vi "HEWH_DSM_CMD.vi"(5 "Temperature":u8=100, 7 "Vacation Days":u8=180, 8 "Heating Mode":T1, 9 "GEA2 Commands and Requests":T2=enum."CMD_WRITE_SETPOINTS") -> (1 "CMD Array":u8[](array[numeric]) format="%x", 2 "Input Data":T5 {"Command" format="%02x"; "Destination" format="%02x"; "Source" format="%02x"})   [LabVIEW 2016]
uses:
  LabVIEW GEA2 Toolkit v1.0.0.0/type defs/Data In.ctl
  Type Definitions/GEA2 Commands.ctl
  Save File/File Setup (Public)/Type Definition/Save File HEWH Heating Control Mode.ctl
  LabVIEW GEA2 Toolkit v1.0.0.0/library/GEA2_Toolkit.lvlib
  Save File/File Setup.lvlib
panel:
  out "element":T3 {"CMD Array" format="%x"; "Destination" format="%x"}
  out "GEA2 Command Cluster":T4(array[cluster])
  out "GEA2 Command Table":string[][](array[string])=[["CMD_WRITE_SETPOINTS", "0x60", "0xA5", "N/A", "Any"], ["RQST_NON_CRIT_VERSION", "0x60", "0x01", "N/A", "Any"], ["RQST_CRIT_VERSION", "0x60", "0x02", "N/A", "Any"], ["RQST_EEPROM_VERSION", "0x60", "0x03", "N/A", "Any"], ["RQST_T2_RESISTANCE", "0x60", "0x10", "N/A", "Any"], ["RQST_T3A_RESISTANCE", "0x60", "0x11", "N/A", "Any"], ["RQST_T3B_RESISTANCE", "0x60", "0x12", "N/A", "Any"], ["RQST_T4_RESISTANCE", "0x60", "0x13", "N/A", "Any"], ["RQST_T5_RESISTANCE", "0x60", "0x14", "N/A", "Any"], ["RQST_IDLB_RESISTANCE", "0x60", "0x15", "N/A", "Any"], ["RQST_MODE_SELECT_RESISTANCE", "0x60", "0x16", "N/A", "Any"], ["RQST_STATUS INFO", "0x60", "0x50", "N/A", "Any"], ["RQST_SS_FAULT_COUNTS", "0x60", "0x53", "N/A", "Any"], ["RQST_OTHER_FAULT_COUNTS", "0x60", "0x54", "N/A", "Any"], ["CMD_CLEAR_FAULT_COUNTS", "0x60", "0x55", "N/A", "Any"], ["RQST_HYPERTERM_OUTPUT_DATA", "0x60", "0x56", "N/A", "Any"], ["RQST_READ_PERSONALITY", "0x60", "0xBC", "N/A", "Any"], ["RQST_DSM_OVERRIDE_STATUS", "0x60", "0xDE", "0x02", "Any"], ["RQST_STATUS_QUERY", "0x60", "0xDE", "0x10", "Any"], ["RQST_HEM_KWH_DATA", "0x60", "0xDE", "0x12", "Any"], ["RQST_SERVICE_ERROR_CODES", "0x60", "0xDE", "0x14", "Any"], ["RQST_OVERRIDE_STATUS", "0x60", "0xDE", "0x17", "Any"], ["CMD_CLEAR_OVERRIDE_STATUS", "0x60", "0xDF", "0x03", "0x40"], ["CMD_CLEAR_ENERGY_USAGE_CTRS", "0x60", "0xDF", "0x07", "0x40"], ["CMD_COMP_OFF", "0x60", "0xF0", "N/A", "Any"], ["CMD_UE_2_SECONDS", "0x60", "0xF3", "N/A", "Any"], ["CMD_LE_2_SECONDS", "0x60", "0xF4", "N/A", "Any"], ["CMD_COMP_ON", "0x60", "0xF5", "N/A", "Any"], ["CMD_HP_RUN_6MIN", "0x60", "0xF6", "N/A", "Any"], ["RQST_TEMP_RANGE", "0x60", "0xF7", "N/A", "Any"], ["RQST_VACATION_RANGE", "0x60", "0xF8", "N/A", "Any"], ["RQST_STD_ELEC_RANGE", "0x60", "0xF9", "N/A", "Any"], ["RQST_WATER_CAPACITY", "0x60", "0xFA", "N/A", "Any"], ["CMD_CANCEL_EEV_POSITION", "0x60", "0xFB", "N/A", "Any"], ["RQST_SUPPORTED_MODES", "0x60", "0xFE", "N/A", "Any"], ["CMD_CONTROL_FAN1", "0x60", "0xF1", "N/A", "Any"], ["CMD_EEV_POSITION", "0x60", "0xFC", "N/A", "Any"], ["CMD_SET_EEV_START_POSITION", "0x60", "E5", "N/A", "Any"], ["CMD_SET_EEV_STOP_POSITION", "0x60", "EA", "N/A", "Any"], ["CMD_UPDATE_DSM_LEVEL", "0x60", "0xDF", "0x00", "0x40"], ["CMD_SET_PID_I_DENOMINATOR", "0x60", "E3", "N/A", "Any"], ["CMD_SET_PID_I_NUMERATOR", "0x60", "E2", "N/A", "Any"], ["RQST_DATA_FROM_MEMORY", "0x60", "0x4E", "N/A", "Any"], ["CMD_OVERRIDE_STATUS_CHANGED", "0x40", "0xDF", "0x02", "0x60"], ["CMD_SET_PID_P_DENOMINATOR", "0x60", "E1", "N/A", "Any"], ["CMD_SET_PID_P_NUMERATOR", "0x60", "E0", "N/A", "Any"], ["CMD_SET_PID_RUN_SH_TARGET", "0x60", "E9", "N/A", "Any"], ["CMD_SET_PID_START_DWELL_TIME", "0x60", "E6", "N/A", "Any"], ["CMD_SET_PID_TRANSITION_TIME", "0x60", "E8", "N/A", "Any"], ["CMD_SET_PID_TRANS_SH_TARGET", "0x60", "E7", "N/A", "Any"], ["CMD_SET_PID_UPDATE_RATE", "0x60", "E4", "N/A", "Any"], ["RQST_DATA_FROM_DATA_FLASH", "0x60", "0x4F", "N/A", "Any"], ["CMD_DSM_OVERRIDES", "0x60", "0xDF", "0x13", "Any"], ["CMD_UPDATE_MODE", "0x60", "0xDF", "0x14", "Any"], ["CMD_UPDATE_SPECIAL_OPERATION", "0x60", "0xDF", "0x15", "Any"], ["CMD_SET_CURRENTS", "0x60", "0xFD", "N/A", "Any"], ["CMD_RESET_FILTER_TIMES", "0x60", "0x90", "N/A", "Any"], ["CMD_TURN_ON_DLB", "0x60", "B0", "N/A", "Any"], ["RQST_PID_PARAMETERS", "0x60", "EF", "N/A", "Any"], ["CMD_CHECK_CRC", "0x60", "0xA6", "N/A", "Any"], ["CMD_ENTER_FACT_MODE", "0x60", "0xC0", "N/A", "Any"], ["CMD_RESET", "0x60", "0xC1", "N/A", "Any"], ["CMD_RESTORE_EEPROM_DEFAULTS", "0x60", "0xC2", "N/A", "Any"], ["RQST_SOFTWARE_VERSION", "0x60", "0x01", "N/A", "0x01"]]
  in  "Tab Control":enum32{"New Parameters"}(tab)
  in  "Source":u8=128 format="%x"
  in  "Input Data 2":T5 {"Command" format="%02x"; "Destination" format="%02x"; "Source" format="%02x"}
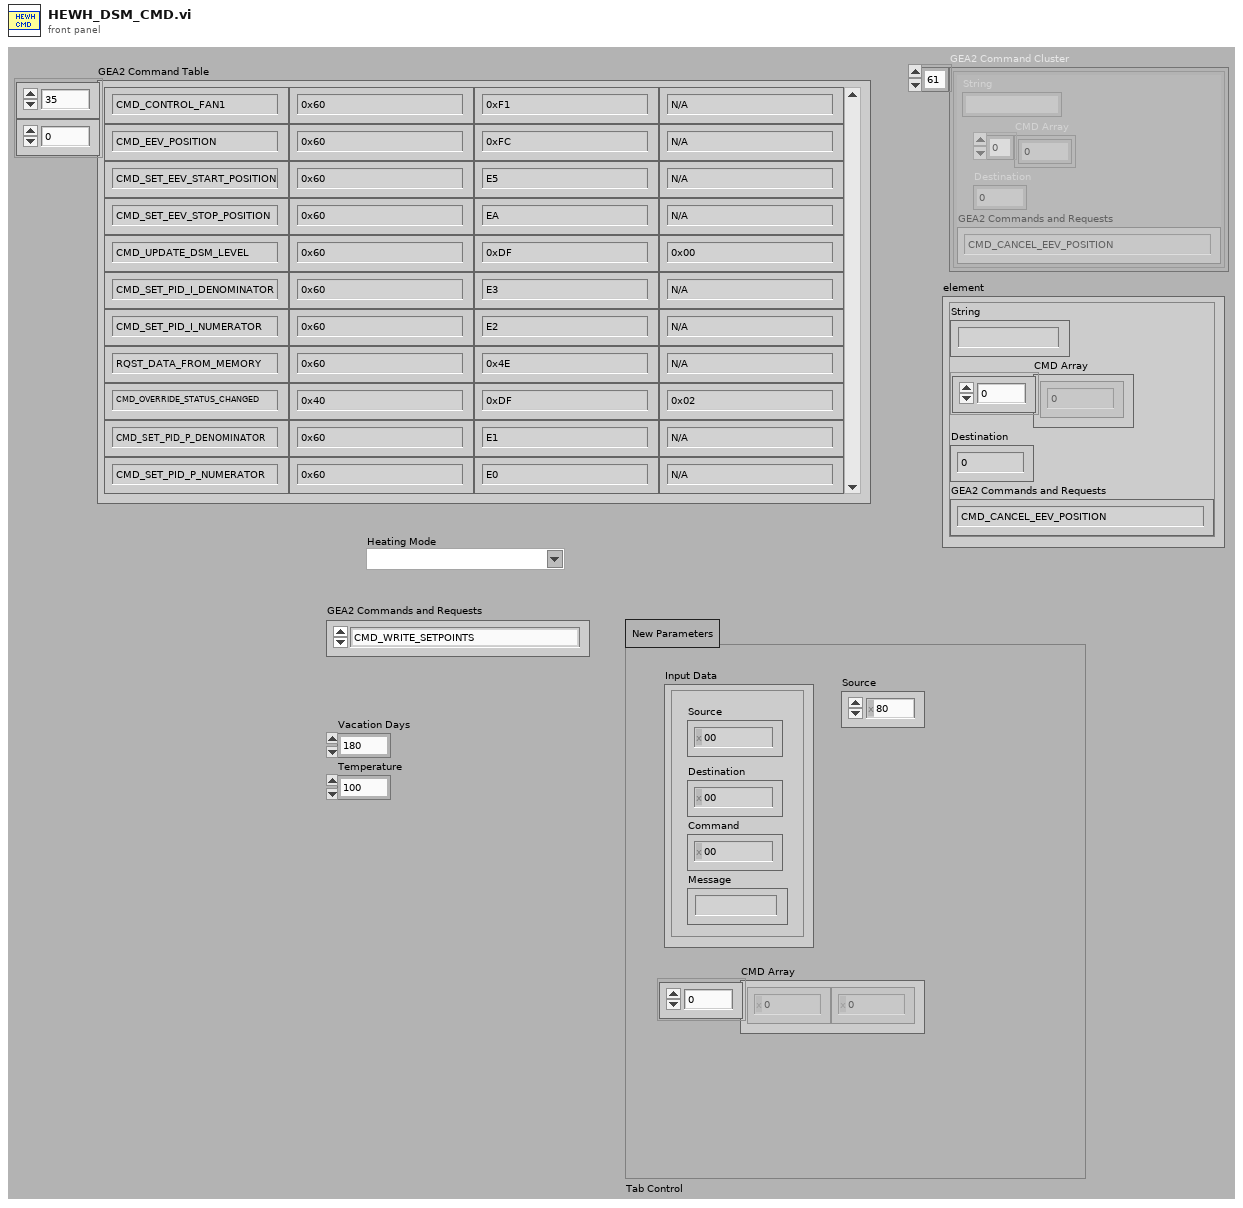
[diagram p1: front panel]
types:
  T1 = typedef "File Setup.lvlib/Save File HEWH Heating Control Mode.ctl" = string
  T2 = typedef "GEA2 Commands.ctl" = enum16{"CMD_CANCEL_EEV_POSITION", "CMD_CLEAR_ENERGY_USAGE_CTRS", "CMD_CLEAR_FAULT_COUNTS", "CMD_CLEAR_OVERRIDE_STATUS", "CMD_COMP_OFF", "CMD_COMP_ON", "CMD_DSM_OVERRIDES", "CMD_EEV_POSITION", "CMD_ENTER_EXIT_FCT_MODE", "CMD_ENTER_FACT_MODE", "CMD_HP_RUN_6MIN", "CMD_INITIATE_REMOTE_DSM_OVERRIDE", "CMD_LE_2_SECONDS", "CMD_REFRESH_SERVICE_TIMEOUTS", "CMD_RESET", "CMD_RESET_FILTER_TIMES", "CMD_RESTORE_EEPROM_DEFAULTS", "CMD_RQST_LED_STATUS", "CMD_SET_AMBIENT_THRESH_1", "CMD_SET_AMBIENT_THRESH_2", "CMD_SET_AMBIENT_THRESH_3", "CMD_SET_CURRENTS", "CMD_SET_EEV_DRIVE_LINES", "CMD_SET_EEV_STOP_POSITION", "CMD_SET_LEDS", "CMD_SET_MODEL_NUMBER", "CMD_SET_PID_I_DENOM_OVER_THR", "CMD_SET_PID_I_DENOM_UNDER_THR", "CMD_SET_PID_LOW_SH_TARGET", "CMD_SET_PID_MID_SH_TARGET", "CMD_SET_PID_P_DENOMINATOR", "CMD_SET_SERIAL_NUMBER", "CMD_SET_START_POS_OVER_THR", "CMD_SET_START_POS_UNDER_THR", "CMD_TOGGLE_FAN", "CMD_TOGGLE_LE_SERV", "CMD_TOGGLE_SERVICE_MODE", "CMD_TOGGLE_UE_SERV", "CMD_TURN_ON_OFF_DLB", "CMD_UE_2_SECONDS", "CMD_UPDATE_DSM_LEVEL", "CMD_UPDATE_MODE", "CMD_WRITE_SETPOINTS", "REQ_READ_KEY_STATUS", "REQ_SYSTEM_MODE", "RQST_CURRENT_PID_SH_TARGET", "RQST_DATA_FROM_DATA_FLASH", "RQST_DATA_FROM_MEMORY", "RQST_DSM_OVERRIDE_STATUS", "RQST_HEM_KWH_DATA", "RQST_HYPERTERM_OUTPUT_DATA", "RQST_IDLB_RESISTANCE", "RQST_MODEL_NUMBER", "RQST_MODEL_SELECT_AD_VALUE", "RQST_OTHER_FAULT_COUNTS", "RQST_OVERRIDE_STATUS", "RQST_PID_PARAMETERS", "RQST_READ_PERSONALITY", "RQST_SERIAL_NUMBER", "RQST_SERVICE_ERROR_CODES", "RQST_Software_Version", "RQST_SS_FAULT_COUNTS", "RQST_STATUS_QUERY", "RQST_STD_ELEC_RANGE", "RQST_SUPPORTED_MODES", "RQST_T2_RESISTANCE", "RQST_T3B_RESISTANCE", "RQST_T4_RESISTANCE", "RQST_T5_RESISTANCE", "RQST_TEMP_RANGE", "RQST_VACATION_RANGE", "RQST_WATER_CAPACITY"}
  T3 = cluster{"String":string, "CMD Array":u8[], "Destination":u8, "GEA2 Commands and Requests":T2}
  T4 = cluster{"String":string, "CMD Array":u8[], "Destination":u8, "GEA2 Commands and Requests":T2}[]
  T5 = typedef "GEA2_Toolkit.lvlib/Data In.ctl" = cluster{"Source":u8, "Destination":u8, "Command":u8, "Message":string}
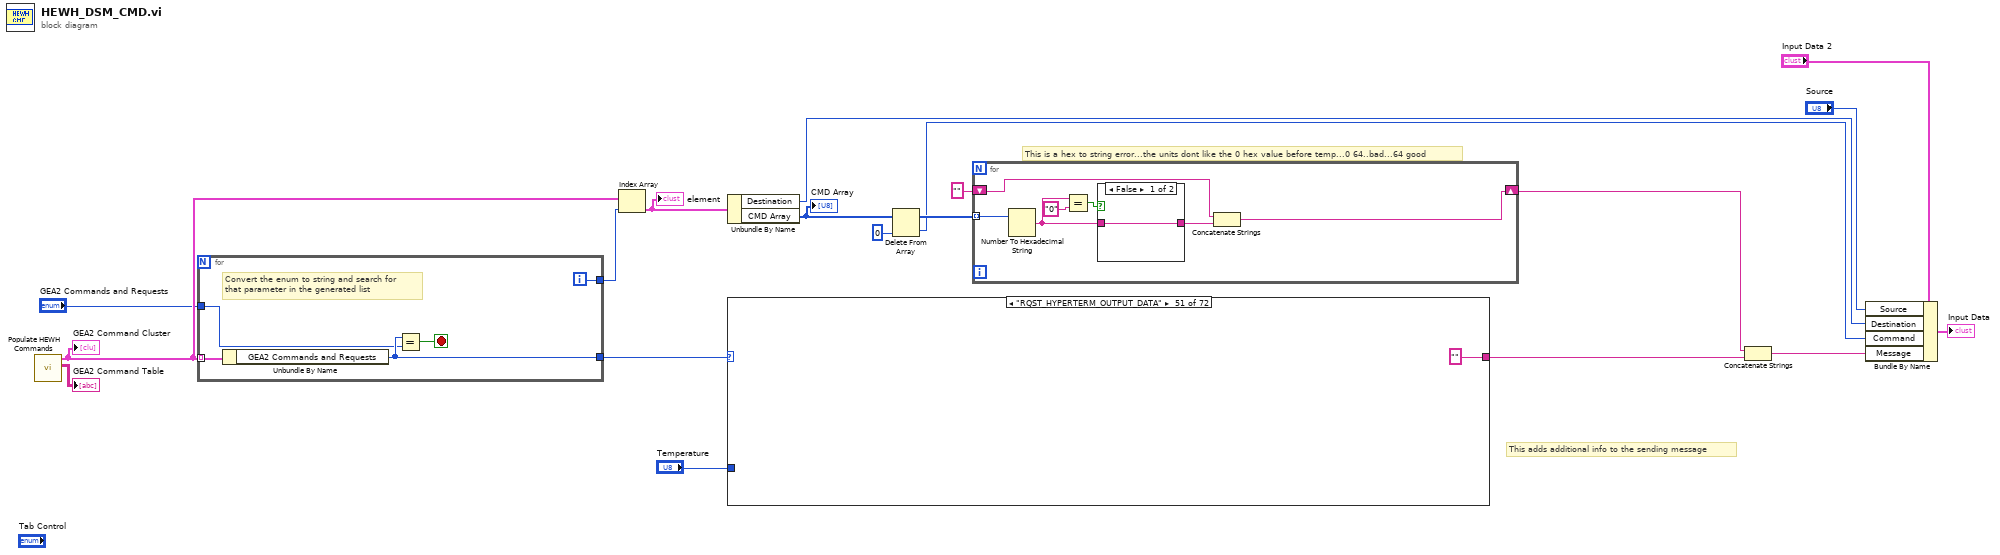
[diagram p0: block diagram]
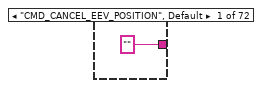
[diagram p2: hidden frame]
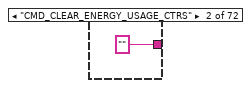
[diagram p3: hidden frame]
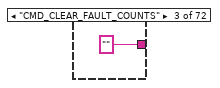
[diagram p4: hidden frame]
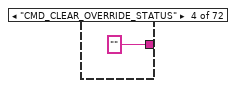
[diagram p5: hidden frame]
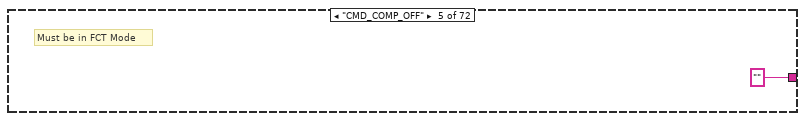
[diagram p6: hidden frame]
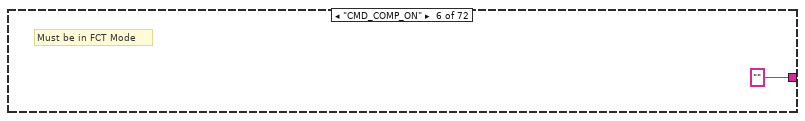
[diagram p7: hidden frame]
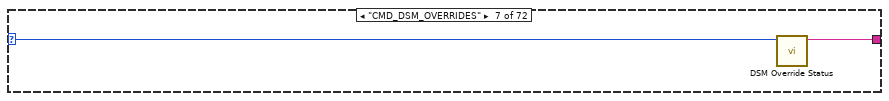
[diagram p8: hidden frame]
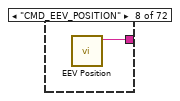
[diagram p9: hidden frame]
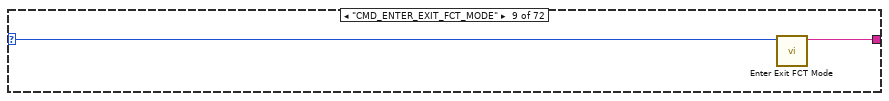
[diagram p10: hidden frame]
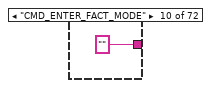
[diagram p11: hidden frame]
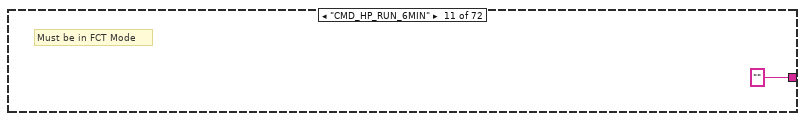
[diagram p12: hidden frame]
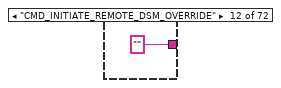
[diagram p13: hidden frame]
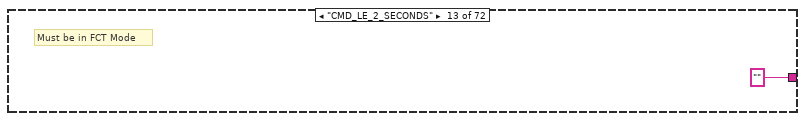
[diagram p14: hidden frame]
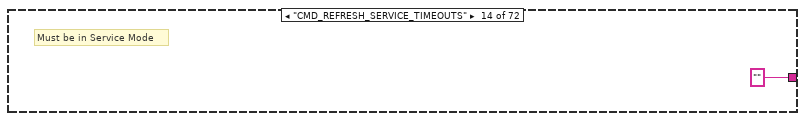
[diagram p15: hidden frame]
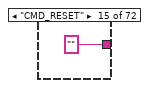
[diagram p16: hidden frame]
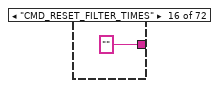
[diagram p17: hidden frame]
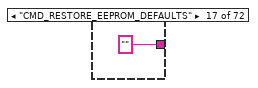
[diagram p18: hidden frame]
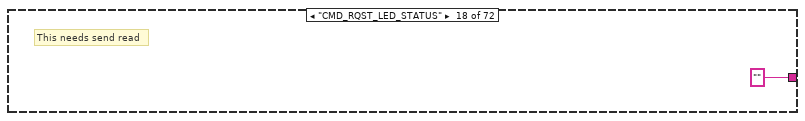
[diagram p19: hidden frame]
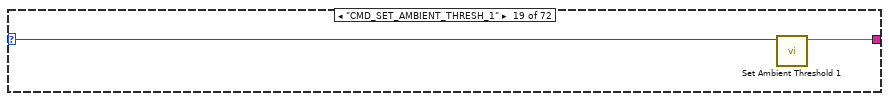
[diagram p20: hidden frame]
diagram:
  # "This is a hex to string error...the units dont like the 0 hex value before temp...0 64..bad...64 good"
  # "This adds additional info to the sending message"
  n1 = call "Populate HEWH Commands.vi"() -> ("GEA2 Command Table"=→"GEA2 Command Table":string[][], "GEA2 Command Cluster"=w5:T4)  [unwired: 10 in]
  "GEA2 Command Cluster" <- w5
  n2 = for {
    tunnel: w5 -> [w24] mode=indexing
    tunnel: [w23] -> w3
    tunnel: "GEA2 Commands and Requests" -> [w22]
    tunnel: [w20] -> w6
    i -> [w20]
    stop <- w21 stop-if-true
    # "Convert the enum to string and search for \nthat parameter in the generated list"
    n3 = Unbundle By Name(w24) -> ("GEA2 Commands and Requests"=w23:T2)
    n4 = Equal?(x=w23, y=w22) -> (x = y?=w21:bool)
  }
  n5 = Index Array(array=w5, index=w6) -> (element=w19:T3)
  "element" <- w19
  n6 = Unbundle By Name(w19) -> ("Destination"=w15:u8, "CMD Array"=w14:u8[])
  "CMD Array" <- w14
  n7 = case shown="\"RQST_HYPERTERM_OUTPUT_DATA\"" w3 {
    selector: w3 -> [_ _ _ _ _ _ w31 _ w34 _ _ _ _ _ _ _ _ _ w45 w47 w49 _ _ _ _ w55 w57 w59 w61 w63 w65 w68 w70 w71 w73 w75 w77 w79 _ _ _ _ _ _ _ _ _ _ _ _ _ _ _ _ _ _ _ _ _ _ _ _ _ _ _ _ _ _ _ _ _ _]
    tunnel: "Temperature" -> [_ _ _ _ _ _ _ _ _ _ _ _ _ _ _ _ _ _ _ _ _ _ _ _ _ _ _ _ _ _ _ _ _ _ _ _ _ _ _ _ _ w89 w103 _ _ _ _ _ _ _ _ _ _ _ _ _ _ _ _ _ _ _ _ _ _ _ _ _ _ _ _ _]
    tunnel: ["" "" "" "" "" "" w32 w33 w35 "" ("DSM Message") "" ("DSM Message") "" ("DSM Message") "" ("DSM Message") "" ("DSM Message") "" ("DSM Message") "" ("DSM Message") "" ("DSM Message") "" ("DSM Message") w46 w48 w50 w51 w52 w53 w54 w56 w58 w60 w62 w64 w66 w67 w69 w72 w74 w76 w78 w80 "" ("DSM Message") "" ("DSM Message") w83 w90 w104 "" ("DSM Message") "" ("DSM Message") "" ("DSM Message") w108 w109 "" ("DSM Message") "" ("DSM Message") "" ("DSM Message") "" ("DSM Message") "" ("DSM Message") "" ("DSM Message") "" ("DSM Message") "" ("DSM Message") "" ("DSM Message") "" ("DSM Message") "" ("DSM Message") "" ("DSM Message") "" ("DSM Message") "" ("DSM Message") "" ("DSM Message") "" ("DSM Message") "" ("DSM Message") "" ("DSM Message") "" ("DSM Message") "" ("DSM Message") "" ("DSM Message") "" ("DSM Message") "" ("DSM Message") "" ("DSM Message")] -> w1
    frame "CMD_CANCEL_EEV_POSITION", Default {
    }
    frame "CMD_CLEAR_ENERGY_USAGE_CTRS" {
    }
    frame "CMD_CLEAR_FAULT_COUNTS" {
    }
    frame "CMD_CLEAR_OVERRIDE_STATUS" {
    }
    frame "CMD_COMP_OFF" {
      # "Must be in FCT Mode"
    }
    frame "CMD_COMP_ON" {
      # "Must be in FCT Mode"
    }
    frame "CMD_DSM_OVERRIDES" {
      n8 = call "DSM Override Status.vi"("Enum"=w31) -> ("DSM Message"=w32:string)  [unwired: 10 in]
    }
    frame "CMD_EEV_POSITION" {
      n9 = call "EEV Position.vi"() -> ("DSM Message"=w33:string)  [unwired: 11 in]
    }
    frame "CMD_ENTER_EXIT_FCT_MODE" {
      n10 = call "Enter Exit FCT Mode.vi"("Enum"=w34) -> ("DSM Message"=w35:string)  [unwired: 10 in]
    }
    frame "CMD_ENTER_FACT_MODE" {
    }
    frame "CMD_HP_RUN_6MIN" {
      # "Must be in FCT Mode"
    }
    frame "CMD_INITIATE_REMOTE_DSM_OVERRIDE" {
    }
    frame "CMD_LE_2_SECONDS" {
      # "Must be in FCT Mode"
    }
    frame "CMD_REFRESH_SERVICE_TIMEOUTS" {
      # "Must be in Service Mode"
    }
    frame "CMD_RESET" {
    }
    frame "CMD_RESET_FILTER_TIMES" {
    }
    frame "CMD_RESTORE_EEPROM_DEFAULTS" {
    }
    frame "CMD_RQST_LED_STATUS" {
      # "This needs send read"
    }
    frame "CMD_SET_AMBIENT_THRESH_1" {
      n11 = call "Set Ambient Threshold 1.vi"("Enum"=w45) -> ("DSM Message"=w46:string)  [unwired: 10 in]
    }
    frame "CMD_SET_AMBIENT_THRESH_2" {
      n12 = call "Set Ambient Threshold 1.vi"("Enum"=w47) -> ("DSM Message"=w48:string)  [unwired: 10 in]
    }
    frame "CMD_SET_AMBIENT_THRESH_3" {
      n13 = call "Set Ambient Threshold 1.vi"("Enum"=w49) -> ("DSM Message"=w50:string)  [unwired: 10 in]
    }
    frame "CMD_SET_CURRENTS" {
      n14 = call "Set Currents.vi"() -> ("DSM Message"=w51:string)  [unwired: 11 in]
    }
    frame "CMD_SET_EEV_DRIVE_LINES" {
      n15 = call "Set EEV Drive Lines.vi"() -> ("DSM Message"=w52:string)  [unwired: 11 in]
    }
    frame "CMD_SET_EEV_STOP_POSITION" {
      n16 = call "EEV Position.vi"() -> ("DSM Message"=w53:string)  [unwired: 11 in]
    }
    frame "CMD_SET_LEDS" {
      # "Must be in FCT Mode"
      n17 = call "Set LEDs.vi"() -> ("DSM Message"=w54:string)  [unwired: 11 in]
    }
    frame "CMD_SET_MODEL_NUMBER" {
      n18 = call "Set Model Number.vi"("Enum"=w55) -> ("DSM Message"=w56:string)  [unwired: 10 in]
    }
    frame "CMD_SET_PID_I_DENOM_OVER_THR" {
      n19 = call "PID Denominator.vi"("Enum"=w57) -> ("DSM Message"=w58:string)  [unwired: 10 in]
    }
    frame "CMD_SET_PID_I_DENOM_UNDER_THR" {
      n20 = call "PID Denominator.vi"("Enum"=w59) -> ("DSM Message"=w60:string)  [unwired: 10 in]
    }
    frame "CMD_SET_PID_LOW_SH_TARGET" {
      n21 = call "Set Ambient Threshold 1.vi"("Enum"=w61) -> ("DSM Message"=w62:string)  [unwired: 10 in]
    }
    frame "CMD_SET_PID_MID_SH_TARGET" {
      n22 = call "Set Ambient Threshold 1.vi"("Enum"=w63) -> ("DSM Message"=w64:string)  [unwired: 10 in]
    }
    frame "CMD_SET_PID_P_DENOMINATOR" {
      n23 = call "PID Denominator.vi"("Enum"=w65) -> ("DSM Message"=w66:string)  [unwired: 10 in]
    }
    frame "CMD_SET_SERIAL_NUMBER" {
      n24 = call "Set Model Number.vi"("Enum"=w68) -> ("DSM Message"=w67:string)  [unwired: 10 in]
    }
    frame "CMD_SET_START_POS_OVER_THR" {
      n25 = call "PID Denominator.vi"("Enum"=w70) -> ("DSM Message"=w69:string)  [unwired: 10 in]
    }
    frame "CMD_SET_START_POS_UNDER_THR" {
      n26 = call "PID Denominator.vi"("Enum"=w71) -> ("DSM Message"=w72:string)  [unwired: 10 in]
    }
    frame "CMD_TOGGLE_FAN" {
      n27 = call "DSM Override Status.vi"("Enum"=w73) -> ("DSM Message"=w74:string)  [unwired: 10 in]
    }
    frame "CMD_TOGGLE_LE_SERV" {
      n28 = call "Enter Exit FCT Mode.vi"("Enum"=w75) -> ("DSM Message"=w76:string)  [unwired: 10 in]
    }
    frame "CMD_TOGGLE_SERVICE_MODE" {
      n29 = call "Enter Exit FCT Mode.vi"("Enum"=w77) -> ("DSM Message"=w78:string)  [unwired: 10 in]
    }
    frame "CMD_TOGGLE_UE_SERV" {
      n30 = call "Enter Exit FCT Mode.vi"("Enum"=w79) -> ("DSM Message"=w80:string)  [unwired: 10 in]
    }
    frame "CMD_TURN_ON_OFF_DLB" {
    }
    frame "CMD_UE_2_SECONDS" {
    }
    frame "CMD_UPDATE_DSM_LEVEL" {
      n31 = call "Update DSM Level.vi"() -> ("DSM Message"=w83:string)  [unwired: 11 in]
    }
    frame "CMD_UPDATE_MODE" {
      # "Stack the messages"
      n32 = case shown="\"Hybrid\"" "Heating Mode" {
        tunnel: [string[] ["10"] string[] ["00"] string[] ["01"] string[] ["02"] string[] ["03"] string[] ["04"]] -> w84
        frame Default {
          # "Dummy value. If its blank i dont want it to change\nmodes. \"10\" is not used"
        }
        frame "Hybrid" {
        }
        frame "Standard" {
        }
        frame "Heat Pump" {
        }
        frame "Boost" {
        }
        frame "Vacation" {
        }
      }
      n33 = Number To Hexadecimal String(2:"Vacation Days") -> (0:w86:string)  [unwired: 1 in]
      n34 = Number To Hexadecimal String(2:w89) -> (0:w87:string)  [unwired: 1 in]
      n35 = Build Array (concatenate)(w84, w86, w87) -> (w91:string[])
      n36 = for {
        tunnel: w91 -> [w99] mode=indexing
        shift-right: [w101] -> w90
        shift-left: "" -> [w102]
        n37 = call <vilib>:"Space Constant.vi"() -> ("String"=w100:string)
        n38 = Concatenate Strings(w102, w100, w99) -> (w101:string)
      }
    }
    frame "CMD_WRITE_SETPOINTS" {
      n39 = Number To Hexadecimal String(2:w103) -> (0:w104:string)  [unwired: 1 in]
    }
    frame "REQ_READ_KEY_STATUS" {
    }
    frame "REQ_SYSTEM_MODE" {
    }
    frame "RQST_CURRENT_PID_SH_TARGET" {
    }
    frame "RQST_DATA_FROM_DATA_FLASH" {
      n40 = call "Request Data From Flash.vi"() -> ("DSM Message"=w108:string)  [unwired: 11 in]
    }
    frame "RQST_DATA_FROM_MEMORY" {
      n41 = call "Data From Memory.vi"() -> ("DSM Message"=w109:string)  [unwired: 11 in]
    }
    frame "RQST_DSM_OVERRIDE_STATUS" {
    }
    frame "RQST_HEM_KWH_DATA" {
    }
    frame "RQST_HYPERTERM_OUTPUT_DATA" {
    }
    frame "RQST_IDLB_RESISTANCE" {
    }
    frame "RQST_MODEL_NUMBER" {
    }
    frame "RQST_MODEL_SELECT_AD_VALUE" {
    }
    frame "RQST_OTHER_FAULT_COUNTS" {
    }
    frame "RQST_OVERRIDE_STATUS" {
    }
    frame "RQST_PID_PARAMETERS" {
    }
    frame "RQST_READ_PERSONALITY" {
    }
    frame "RQST_SERIAL_NUMBER" {
    }
    frame "RQST_SERVICE_ERROR_CODES" {
    }
    frame "RQST_SS_FAULT_COUNTS" {
    }
    frame "RQST_STATUS_QUERY" {
    }
    frame "RQST_STD_ELEC_RANGE" {
    }
    frame "RQST_SUPPORTED_MODES" {
    }
    frame "RQST_Software_Version" {
    }
    frame "RQST_T2_RESISTANCE" {
    }
    frame "RQST_T3B_RESISTANCE" {
    }
    frame "RQST_T4_RESISTANCE" {
    }
    frame "RQST_T5_RESISTANCE" {
    }
    frame "RQST_TEMP_RANGE" {
    }
    frame "RQST_VACATION_RANGE" {
    }
    frame "RQST_WATER_CAPACITY" {
    }
  }
  n42 = Delete From Array(array=w14, index=0) -> (deleted portion=w11:u8, array with subset deleted=w12:u8[])  [unwired: 1 in]
  n43 = for {
    tunnel: w12 -> [w140] mode=indexing
    shift-right: [w138] -> w8
    shift-left: "" -> [w139]
    n44 = Number To Hexadecimal String(2:w140) -> (0:w134:string)  [unwired: 1 in]
    n45 = Equal?(x=w134, y="0") -> (x = y?=w136:bool)
    n46 = case shown="False" w136 {
      tunnel: [w141 ""] -> w135
      tunnel: w134 -> [w141 _]
      frame False {
      }
      frame True {
      }
    }
    n47 = Concatenate Strings(w139, w135) -> (w138:string)
  }
  n48 = Concatenate Strings(w8, w1) -> (w7:string)
  n49 = Bundle By Name(cluster="Input Data 2", "Source"="Source", "Destination"=w15, "Command"=w11, "Message"=w7) -> (→"Input Data":T5)
